vi "DestroyHandle.vi"(8 "error in (no error)":errorcluster caption="错误输入（无错误）", 11 "handle":u64) -> (0 "error out":errorcluster caption="错误输出", 2 "function return":i32)   [LabVIEW 2011, in "MvCameraControl.lvlib"]
doc: "MV_LV_API int __stdcall DestroyHandle( void * handle);"
uses:
  MvCameraControl.lvlib
  MvCameraControl.dll
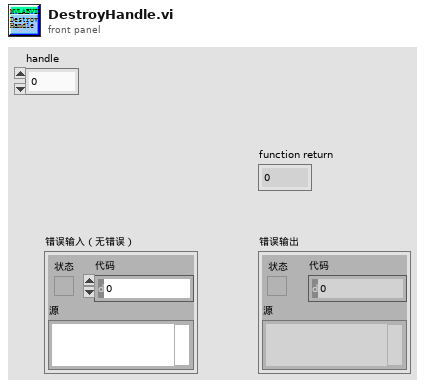
[diagram p1: front panel]
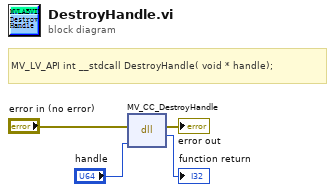
[diagram p0: block diagram]
diagram:
  # "MV_LV_API int __stdcall DestroyHandle( void * handle);"
  n1 = dll-call lib="MvCameraControl.dll" fn="MV_CC_DestroyHandle"(error in="error in (no error)", "handle"="handle") -> (error out=→"error out":errorcluster, "返回类型"=→"function return":i32)  [unwired: 3 in, 1 out]
